vi "RT Main (Cluster Write).vi"() -> ()   [LabVIEW 2018]
uses:
  TypeDefs/Simple cluster.ctl
  58ef3a2b-dcb5-4c85-9d81-a61eb9170448.vi
  09b65eee-4abe-4c0b-8234-30d4a9e3e5f6.vi
  58ef3a2b-dcb5-4c85-9d81-a61eb9170448.vi/24040c1a-84b4-4e70-b997-4a4bb9d358d1.vi
  09b65eee-4abe-4c0b-8234-30d4a9e3e5f6.vi/f3c72d53-d065-40be-9b9a-752fbfdcd54e.vi
  FPGA Bitfile Register Operations/Scalar IO Operations/Utilities/Find Register Offset.vi
  FPGA Bitfile Register Operations/Scalar IO Operations/Utilities/Parser Cluster Configuration.vi
  FPGA Bitfile Register Operations/Scalar IO Operations/Utilities/DBL to FXP.vi
  FPGA Bitfile Register Operations/Scalar IO Operations/Utilities/Convert Bool Array to Cluster BLOB.vi
  FPGA Bitfile Register Operations/Scalar IO Operations/Write Methods/Write U8 Array.vi
  FPGA Bitfile Register Operations/Scalar IO Operations/Read Methods/Read U8 Array.vi
  FPGA Bitfile Register Operations/Scalar IO Operations/Utilities/Convert Cluster BLOB to Bool Array.vi
  FPGA Bitfile Register Operations/Scalar IO Operations/Utilities/FXP to DBL.vi
  <userlib>/_OpenG.lib/lvdata/lvdata.llb/Array of VData to VCluster__ogtk.vi
  <vilib>/FPGAPlugInAG/Dynamic/niLvFpga_Close_Dynamic.vi
  <vilib>/rvi/interface/nirviCloseFPGA/nirviCloseFPGA.xnode
  FPGA Bitfile Register Operations/Scalar IO Operations/Scalar IO Operations.lvlib
panel:
  out "Cluster out":T1
  out "Blob Read":u8[](array[numeric])
  out "BLOB Write":u8[](array[numeric])
  out "Average seconds per read":dbl
  out "error out":errorcluster
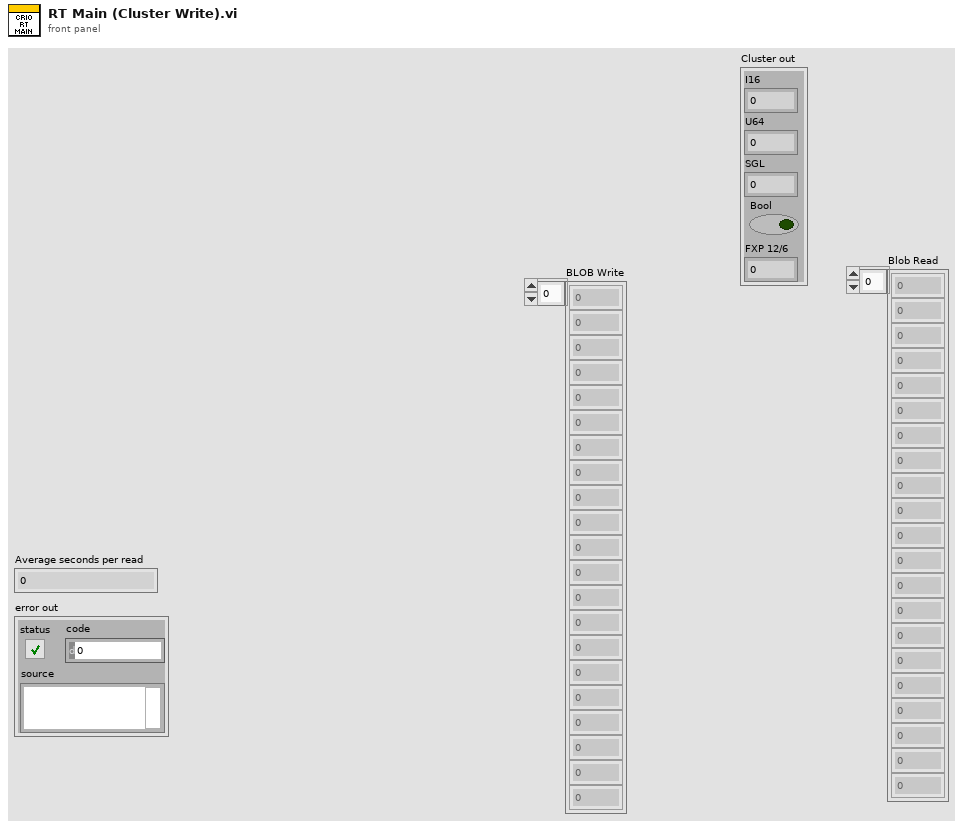
[diagram p1: front panel]
types:
  T1 = typedef "Simple cluster.ctl" = cluster{"I16":i16, "U64":u64, "SGL":sgl, "Bool":bool, "FXP 12/6":fxp<+/-,12,6>}
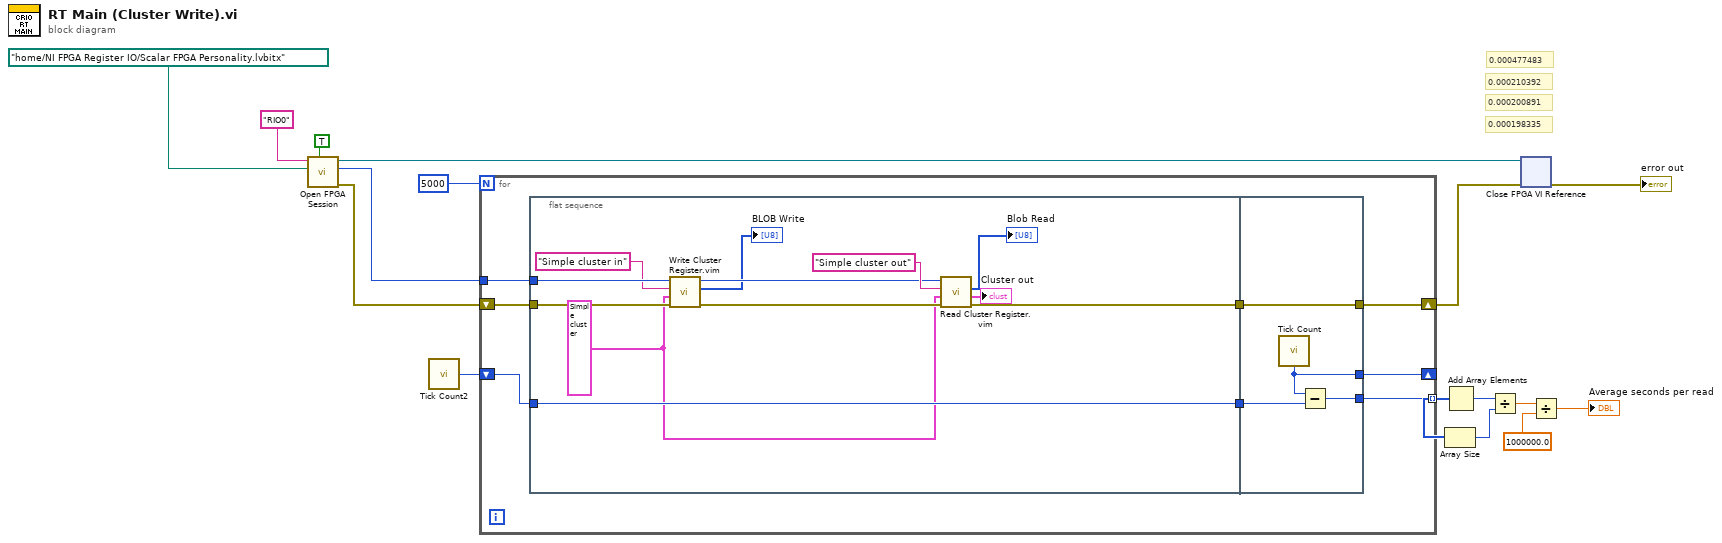
[diagram p0: block diagram]
diagram:
  # "0.000198335"
  # "0.000200891"
  # "0.000210392"
  # "0.000477483"
  n1 = call "Open FPGA Session.vi"("run when loaded (T)"=TRUE ("Run When Loaded (T)"), "bitfile path"=path "/home/NI FPGA Register IO/Scalar FPGA Personality.lvbitx" ("Bitfile path"), "device address"="RIO0" ("Device address")) -> ("error out"=w3:errorcluster, "session out"=w2:u64, "bitfile reference out"=w13:refnum<k20>)  [unwired: 6 in]
  n2 = call "Tick Count2"() -> ("Tick Count(uSec)"=w10:u32)
  n3 = for {
    N: 5000 -> [_]
    shift-right: [w17] -> w1
    shift-left: w3 -> [w24]
    shift-right: [w21] -> _
    shift-left: w10 -> [w23]
    tunnel: [w20] -> w9 mode=indexing
    tunnel: w2 -> [w19]
    n4 = flat-sequence {
      tunnel: w24 -> [w33]
      tunnel: w23 -> [w36]
      tunnel: [w36] -> w22
      tunnel: w19 -> [w34]
      tunnel: [w30] -> w18
      tunnel: w22 -> [w40]
      tunnel: [w39] -> w21
      tunnel: [w38] -> w20
      tunnel: w18 -> [w37]
      tunnel: [w37] -> w17
      frame #0 {
        w27 = T1 {"I16"=0, "U64"=10, "SGL"=10.0, "Bool"=TRUE, "FXP 12/6"=10.0} ("Simple Cluster")
        n5 = call "Write Cluster Register.vim"("error in (no error)"=w33, "Cluster in (default value)"=w27, "Cluster Name"="Simple cluster in" ("register name"), "session in"=w34) -> ("error out"=w32:errorcluster, "Cluster BLOB"=→"BLOB Write":u8[], "session out"=w31:u64)  [unwired: 5 in]
        n6 = call "Read Cluster Register.vim"("error in (no error)"=w32, "Cluster in (default value)"=w27, "Cluster Name"="Simple cluster out" ("register name"), "session in"=w31) -> ("error out"=w30:errorcluster, "Cluster out"=→"Cluster out":T1, "Value out"=→"Blob Read":u8[])  [unwired: 4 in, 1 out]
      }
      frame #1 {
        n7 = call "Tick Count"() -> ("Tick Count(uSec)"=w39:u32)
        n8 = Subtract(x=w39, y=w40) -> (x-y=w38:u32)
      }
    }
  }
  n9 = Array Size(array=w9) -> (size(s)=w7:i32)
  n10 = Add Array Elements(numeric array=w9) -> (sum=w8:u32)
  n11 = Divide(x=w8, y=w7) -> (x/y=w6:dbl)
  n12 = xnode "Close FPGA VI Reference"("FPGA VI Reference In"=w13, "error in"=w1) -> ("error out"=→"error out":errorcluster)
  n13 = Divide(x=w6, y=1000000.0) -> (x/y=→"Average seconds per read":dbl)
